vi "Read 02-03-9227.vi"() -> (3 "02-03-9227":dbl[](array[numeric]))   [LabVIEW 2018, in "Inputs.lvlib"]
uses:
  Inputs.lvlib
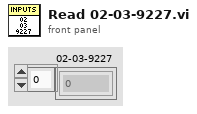
[diagram p1: front panel]
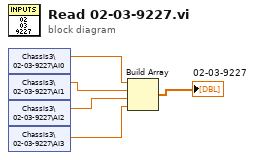
[diagram p0: block diagram]
diagram:
  n1 = shared-variable "Chassis3\\02-03-9227\\AI0"() -> (w2:dbl)  [unwired: 1 in, 1 out]
  n2 = shared-variable "Chassis3\\02-03-9227\\AI1"() -> (w3:dbl)  [unwired: 1 in, 1 out]
  n3 = shared-variable "Chassis3\\02-03-9227\\AI2"() -> (w4:dbl)  [unwired: 1 in, 1 out]
  n4 = shared-variable "Chassis3\\02-03-9227\\AI3"() -> (w5:dbl)  [unwired: 1 in, 1 out]
  n5 = Build Array(w2, w3, w4, w5) -> (→"02-03-9227":dbl[])
